vi "ws_editscenario Load Scenario.vi"(6 "User Information":T2, 7 "command (\"edit\")":string="edit", 8 "error in (no error)":errorcluster, 9 "UploadedFilesList":T1(array[cluster]), 10 "sxScenarioId (\"\")":string, 11 "Connection Refnum":T4) -> (0 "error out":errorcluster, 1 "Template Keys":T3, 2 "sxScenarioId":string, 3 "Connection Refnum":T4, 5 "PREVSCENARIOS array":string)   [LabVIEW 2011]
uses:
  SI.LIB/ODBC/SQL Controls/Connection Refnum.ctl
  <vilib>/addons/internet/utils/keyedarr.llb/Keyed Array.ctl
  server/database/Users/User Record.ctl
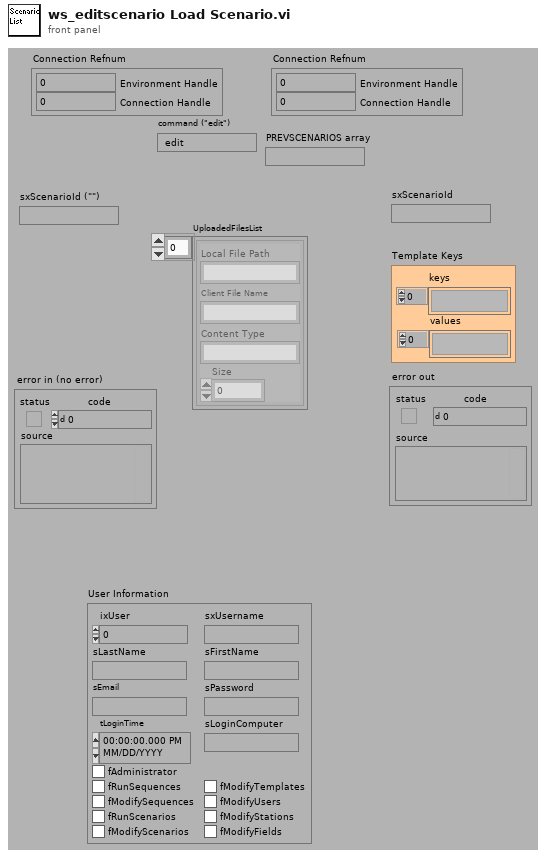
[diagram p1: front panel]
types:
  T1 = cluster{"Local File Path":string, "Client File Name":string, "Content Type":string, "Size":u32}[]
  T2 = typedef "User Record.ctl" = cluster{"ixUser":i32, "sxUsername":string, "sLastName":string, "sFirstName":string, "sEmail":string, "sPassword":string, "tLoginTime":timestamp, "sLoginComputer":string, "fAdministrator":bool, "fRunSequences":bool, "fModifySequences":bool, "fRunScenarios":bool, "fModifyScenarios":bool, "fModifyTemplates":bool, "fModifyUsers":bool, "fModifyStations":bool, "fModifyFields":bool}
  T3 = typedef "Keyed Array.ctl" = cluster{"keys":string[], "values":string[]}
  T4 = typedef "Connection Refnum.ctl" = cluster{"Environment Handle":i32, "Connection Handle":i32}
  T5 = typedef "Scenario Record.ctl" = cluster{"ixScenario":i32, "tCreated":timestamp, "tModified":timestamp, "sxUsername":string, "sModifiedBy":string, "sxScenarioId":string, "sDescription":string, "sLogic":string, "sResultFieldsCSV":string, "sTemplatesCSV":string, "fAutoRunReports":bool, "fSortByTemplates":bool, "fCombinePDF":bool, "Conditions":T6[]}
  T6 = typedef "Condition Record.ctl" = cluster{"iConditionIndex":i32, "sxFieldId":string, "nOperator":T7, "sMatchValue":string}
  T7 = typedef "Condition Operators.ctl" = enum16{"equal (=)", "not equal (\\u2260)", "less than (<)", "less than or equal (\\u2264)", "greater than (>)", "greater than or equal (\\u2265)", "contains", "does not contain"}
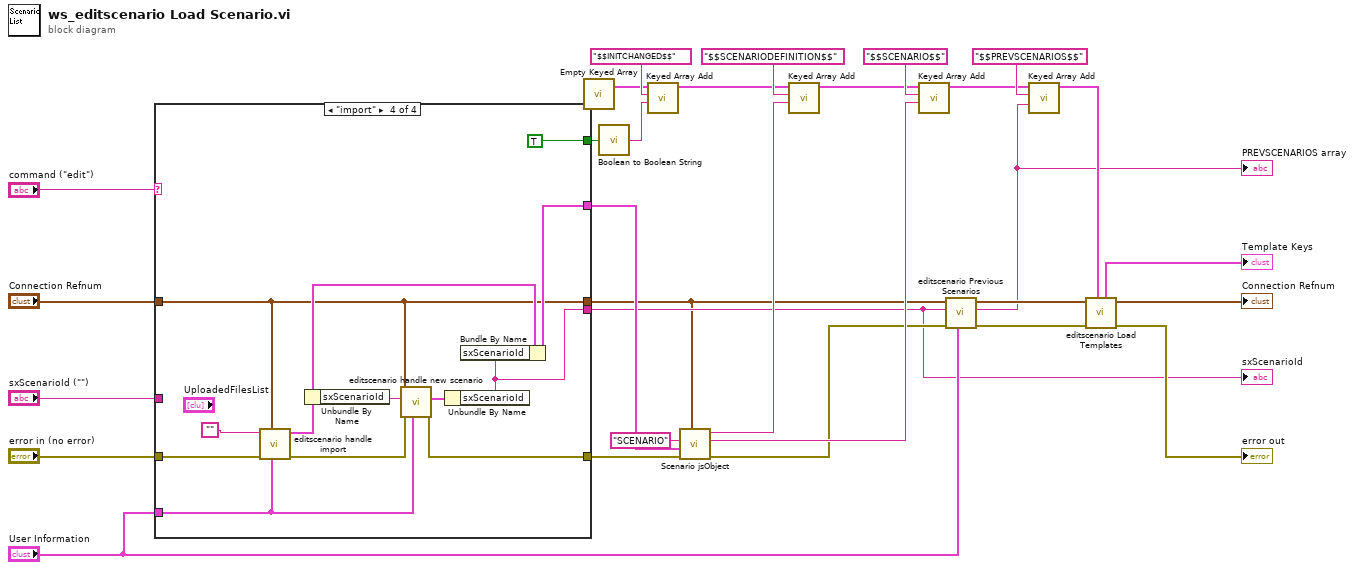
[diagram p0: block diagram]
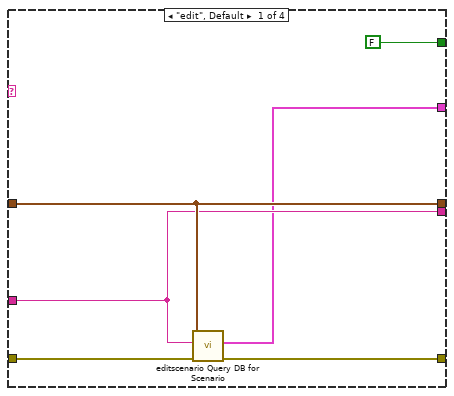
[diagram p2: hidden frame]
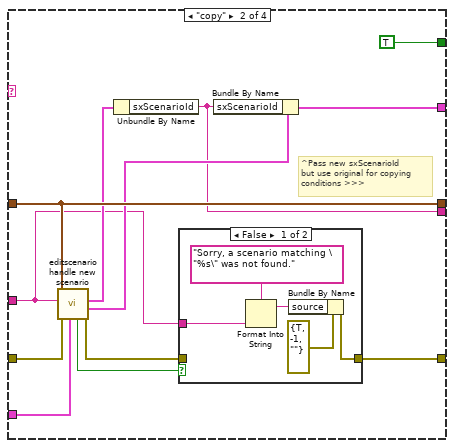
[diagram p3: hidden frame]
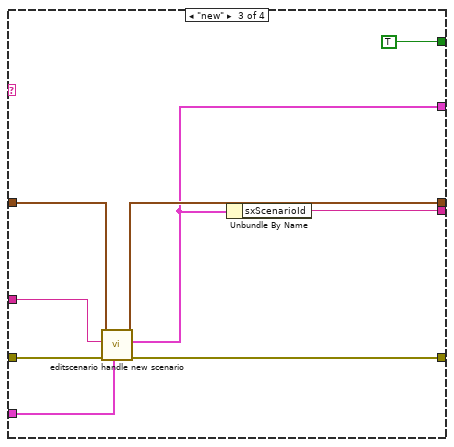
[diagram p5: hidden frame]
diagram:
  n1 = case shown="\"import\"" "command (\"edit\")" {
    tunnel: [w34 w48 w58 w71] -> w11
    tunnel: "sxScenarioId (\"\")" -> [w32 w38 w55 _]
    tunnel: "error in (no error)" -> [w35 w46 w62 w65]
    tunnel: "Connection Refnum" -> [w33 w43 w60 w66]
    tunnel: [w33 w43 w59 w66] -> w1
    tunnel: "User Information" -> [_ w41 w61 w73]
    tunnel: [FALSE TRUE TRUE TRUE] -> w23
    tunnel: [w31 w39 w57 w68] -> w15
    tunnel: [w32 w37 w56 w69] -> w3
    frame "edit", Default {
      n2 = call "editscenario Query DB for Scenario.vi"("error in (no error)"=w35, "sxScenarioId (\"\")"=w32, "Connection Refnum"=w33) -> ("error out"=w34:errorcluster, "Scenario Record"=w31:T5)  [unwired: 7 out]
    }
    frame "copy" {
      # "^Pass new sxScenarioId\nbut use original for copying\nconditions >>>"
      n3 = call "editscenario handle new scenario.vi"("User Information"=w41, "error in (no error)"=w46, "New Name Suggestion\n(empty - \"Username Sequence N\")"=w38, "Connection Refnum"=w43) -> ("error out"=w44:errorcluster, "First Matching Scenario Record"=w42:T5, "New Scenario Record"=w40:T5, "Existed?"=w45:bool)  [unwired: 4 out]
      n4 = Unbundle By Name(w40) -> ("sxScenarioId"=w37:string)
      n5 = case shown="False" w45 {
        tunnel: w44 -> [_ w54]
        tunnel: [w50 w54] -> w48
        tunnel: w38 -> [w49 _]
        frame False {
          n6 = Format Into String(format string="Sorry, a scenario matching \"%s\" was not found.", w49) -> (resulting string=w52:string)  [unwired: 2 in, 1 out]
          n7 = Bundle By Name(cluster=errorcluster {"status"=TRUE, "code"=-1, "source"=""} ("error out"), "source"=w52) -> (w50:errorcluster)
        }
        frame True {
        }
      }
      n8 = Bundle By Name(cluster=w42, "sxScenarioId"=w37) -> (w39:T5)
    }
    frame "new" {
      n9 = call "editscenario handle new scenario.vi"("User Information"=w61, "error in (no error)"=w62, "New Name Suggestion\n(empty - \"Username Sequence N\")"=w55, "Connection Refnum"=w60) -> ("error out"=w58:errorcluster, "New Scenario Record"=w57:T5, "Connection Refnum"=w59:T4)  [unwired: 5 out]
      n10 = Unbundle By Name(w57) -> ("sxScenarioId"=w56:string)
    }
    frame "import" {
      n11 = call "editscenario handle import.vi"("User Information"=w73, "Connection Refnum"=w66, "error in (no error)"=w65, "Scenario XML (\"\")"="") -> ("error out"=w74:errorcluster, "Scenario Record"=w67:T5)  [unwired: 1 in, 5 out]
      n12 = Unbundle By Name(w67) -> ("sxScenarioId"=w72:string)
      n13 = call "editscenario handle new scenario.vi"("User Information"=w73, "error in (no error)"=w74, "New Name Suggestion\n(empty - \"Username Sequence N\")"=w72, "Connection Refnum"=w66) -> ("error out"=w71:errorcluster, "New Scenario Record"=w70:T5)  [unwired: 6 out]
      n14 = Unbundle By Name(w70) -> ("sxScenarioId"=w69:string)
      n15 = Bundle By Name(cluster=w67, "sxScenarioId"=w69) -> (w68:T5)
    }
  }
  "sxScenarioId" <- w3
  n16 = call "Empty Keyed Array.vi"() -> ("empty keyed array"=w2:T3)  [unwired: 3 out]
  n17 = call "Boolean to Boolean String.vi"("Boolean"=w23) -> ("Boolean string"=w24:string)  [unwired: 1 in]
  n18 = call <vilib>:"Keyed Array Add.vi"("value"=w24, "key"="$$INITCHANGED$$", "array in"=w2) -> ("array out"=w17:T3)  [unwired: 2 in, 2 out]
  n19 = call "Scenario jsObject.vi"("Connection Refnum"=w1, "error in (no error)"=w11, "Scenario Record (empty)"=w15, "Scenario jsObject Name (\"\")"="SCENARIO" ("Scenario jsObject Name (\"\")")) -> ("error out"=w6:errorcluster, "Scenario jsObject"=w13:string, "SCENARIO jsObject Definition"=w14:string)  [unwired: 2 in, 3 out]
  n20 = call <vilib>:"Keyed Array Add.vi"("value"=w14, "key"="$$SCENARIODEFINITION$$", "array in"=w17) -> ("array out"=w16:T3)  [unwired: 2 in, 2 out]
  n21 = call <vilib>:"Keyed Array Add.vi"("value"=w13, "key"="$$SCENARIO$$", "array in"=w16) -> ("array out"=w9:T3)  [unwired: 2 in, 2 out]
  n22 = call "editscenario Previous Scenarios.vi"("User Information"="User Information", "error in (no error)"=w6, "sxScenarioId (\"\")"=w3, "Connection Refnum"=w1) -> ("error out"=w7:errorcluster, "Previous SCENARIOS array"=w4:string, "Connection Refnum"=w5:T4)  [unwired: 1 in, 4 out]
  "PREVSCENARIOS array" <- w4
  n23 = call <vilib>:"Keyed Array Add.vi"("value"=w4, "key"="$$PREVSCENARIOS$$", "array in"=w9) -> ("array out"=w8:T3)  [unwired: 2 in, 2 out]
  n24 = call "editscenario Load Templates.vi"("Template Keys (empty)"=w8, "error in (no error)"=w7, "Connection Refnum"=w5) -> ("error out"=→"error out":errorcluster, "Connection Refnum"=→"Connection Refnum":T4, "Template Keys"=→"Template Keys":T3)  [unwired: 6 out]
